vi "Read Data.vi"(6 "NoStop (F)":bool, 8 "error in (no error)":errorcluster, 9 "Len":u8, 11 "I2C Peripheral":refnum<class "I2C Connection.lvclass">) -> (0 "error out":errorcluster, 1 "Data":string)   [LabVIEW 2020, in "CTI.lvlib" / "I2C Connection.lvclass"]
uses:
  I2C Connection.lvclass
  I2C Connection.lvclass/I2C Connection.ctl
  Session/Session.lvclass
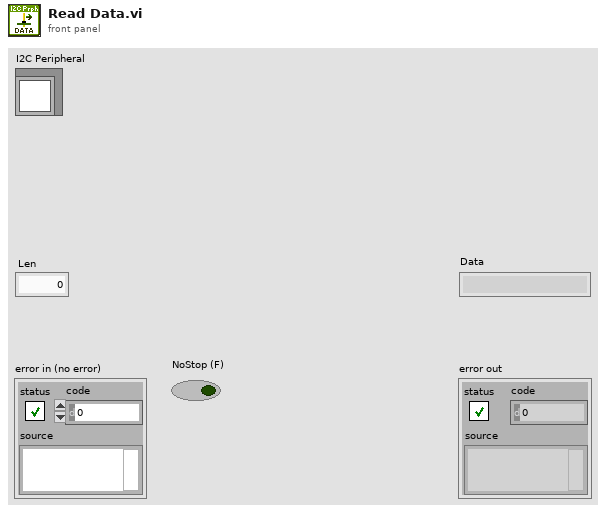
[diagram p1: front panel]
types:
  T1 = typedef "CTI.lvlib/I2C Address.ctl" = u8
  T2 = typedef "CTI.lvlib/I2C Number.ctl" = i8
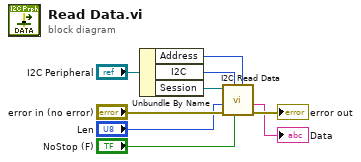
[diagram p0: block diagram]
diagram:
  n1 = Unbundle By Name("I2C Peripheral") -> ("Address"=w4:T1, "I2C"=w5:T2, "Session"=w1:refnum<class "Session.lvclass">)
  n2 = call "I2C Read Data.vi"("Address"=w4, "NoStop (F)"="NoStop (F)", "I2C #"=w5, "error in (no error)"="error in (no error)", "Len"="Len", "Session in"=w1) -> ("error out"=→"error out":errorcluster, "Data"=→"Data":string)  [unwired: 3 in, 1 out]
